vi "Start Trigger Delay.vi"(6 "Seconds":i32, 8 "error in (no error)":errorcluster, 9 "Minutes":i32, 10 "Hours":i32, 11 "VISA resource name":refnum<visa-resource-name>) -> (0 "error out":errorcluster, 3 "VISA resource name out":refnum<visa-resource-name>)   [LabVIEW 2017, in "Sefram DAS220.lvlib"]
doc: "Set start trigger in delay mode : wait for the delay specified before starting recording."
uses:
  <instrlib>/Sefram DAS220/Sefram DAS220.lvlib
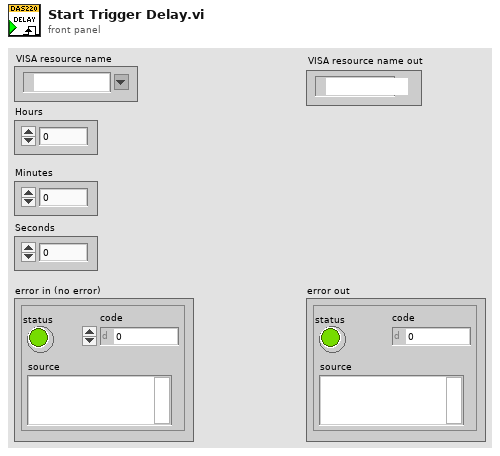
[diagram p1: front panel]
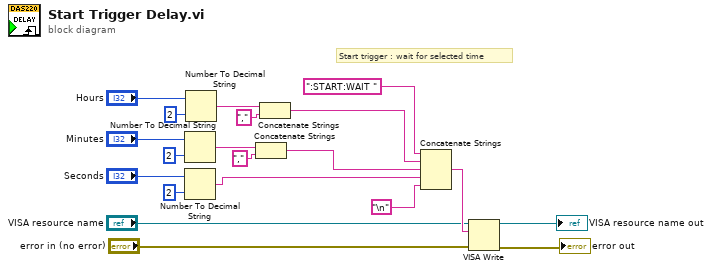
[diagram p0: block diagram]
diagram:
  # "Start trigger : wait for selected time"
  n1 = Number To Decimal String(number="Minutes", width (-)=i16 2) -> (decimal integer string=w4:string)
  n2 = Number To Decimal String(number="Seconds", width (-)=i16 2) -> (decimal integer string=w1:string)
  n3 = Number To Decimal String(number="Hours", width (-)=i16 2) -> (decimal integer string=w7:string)
  n4 = Concatenate Strings(w4, "," ("string")) -> (w2:string)
  n5 = Concatenate Strings(w7, "," ("string")) -> (w5:string)
  n6 = Concatenate Strings(":START:WAIT " ("string"), w5, w2, w1, "\n") -> (w20:string)
  n7 = VISA Write(VISA resource name="VISA resource name", write buffer=w20, error in (no error)="error in (no error)") -> (VISA resource name out=→"VISA resource name out":refnum<visa-resource-name>, error out=→"error out":errorcluster)  [unwired: 1 out]
